vi "Example_MoveToRelativePosition.vi"() -> ()   [LabVIEW 2018]
doc: "Example how to do a relative position step. Before starts this example the device must be tuned and the parameter settings must be correct.\nThe example shows:\n - how to initialise and close an interface (e.g. RS232)\n - start of a positioning with correct operation mode\n - wait until the target position is reached"
panel:
  in  "timeout":u32=1000
  in  "relative position":i32=100
  in  "position profile":T1={"profileVelocity"=1000, "profileAcceleration"=10000, "profileDeceleration"=10000}
  in  "nodeId":u16=1
  in  "communication settings in":T2={"deviceName"="EPOS2", "protocolStackName"="MAXON SERIAL V2", "interfaceName"="USB", "portName"="USB0", "baudrate"=1000000, "timeout"=500}
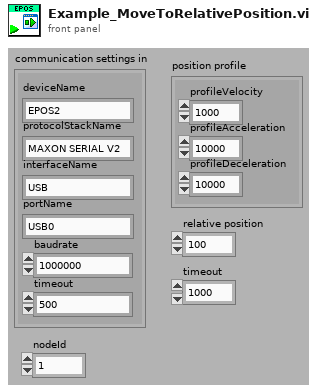
[diagram p1: front panel]
types:
  T1 = cluster{"profileVelocity":u32, "profileAcceleration":u32, "profileDeceleration":u32}
  T2 = cluster{"deviceName":string, "protocolStackName":string, "interfaceName":string, "portName":string, "baudrate":u32, "timeout":u32}
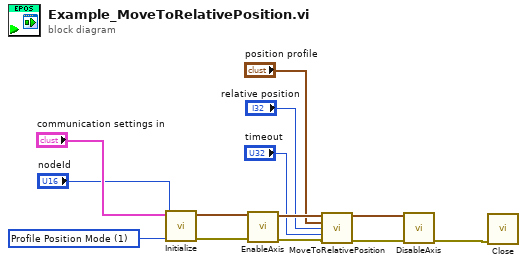
[diagram p0: block diagram]
diagram:
  w12 = i8 1 items=["Profile Position Mode"=1, "Profile Velocity Mode"=3, "Homing Mode"=6, "Interpolated Position Mode"=7, "Position Mode"=-1, "Velocity Mode"=-2, "Current Mode"=-3, "Master Encoder Mode"=-5, "Step Direction Mode"=-6] ("modes of operations")
  n1 = call "Initialize.vi"("modes of operations"=w12, "nodeId"="nodeId", "communication settings in"="communication settings in") -> ("error out"=w10:errorcluster, "axis out"=w7:cluster{"keyHandle":u32, "nodeId":u16})  [unwired: 7 in]
  n2 = call "EnableAxis.vi"("error in (no error)"=w10, "axis in"=w7) -> ("error out"=w9:errorcluster, "axis out"=w6:cluster{"keyHandle":u32, "nodeId":u16})  [unwired: 4 in]
  n3 = call "MoveToRelativePosition.vi"("axis in"=w6, "position profile"="position profile", "relative position"="relative position", "timeout"="timeout", "error in (no error)"=w9) -> ("axis out"=w5:cluster{"keyHandle":u32, "nodeId":u16}, "error out"=w8:errorcluster)  [unwired: 9 in]
  n4 = call "DisableAxis.vi"("error in (no error)"=w8, "axis in"=w5) -> ("error out"=w1:errorcluster)  [unwired: 4 in, 1 out]
  n5 = call "Close.vi"("error in (no error)"=w1) -> ()  [unwired: 10 in, 1 out]
